vi "celsius_to_kelvin.vi"(1 "°C":dbl) -> (0 "K":dbl)   [LabVIEW 2017]
doc: "Convertisseur de °C vers K (°C + 273,15)"
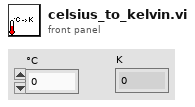
[diagram p1: front panel]
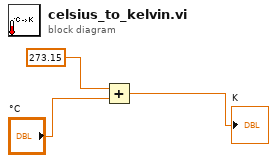
[diagram p0: block diagram]
diagram:
  n1 = Add(x=273.15, y="°C") -> (x+y=→"K":dbl)
